vi "Exercise_3-9_Liam_Hubbard.vi"() -> ()   [LabVIEW 2014]
panel:
  in  "Max Wind Speed":dbl
  in  "Current Wind Speed":dbl
  in  "Current Temp":dbl
  in  "Max Temp":dbl
  in  "Min Temp":dbl
  out "Warning Text":string
  out "Warning?":bool
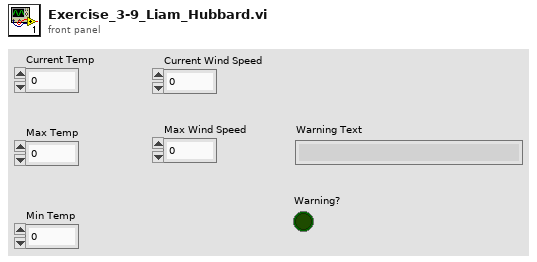
[diagram p1: front panel]
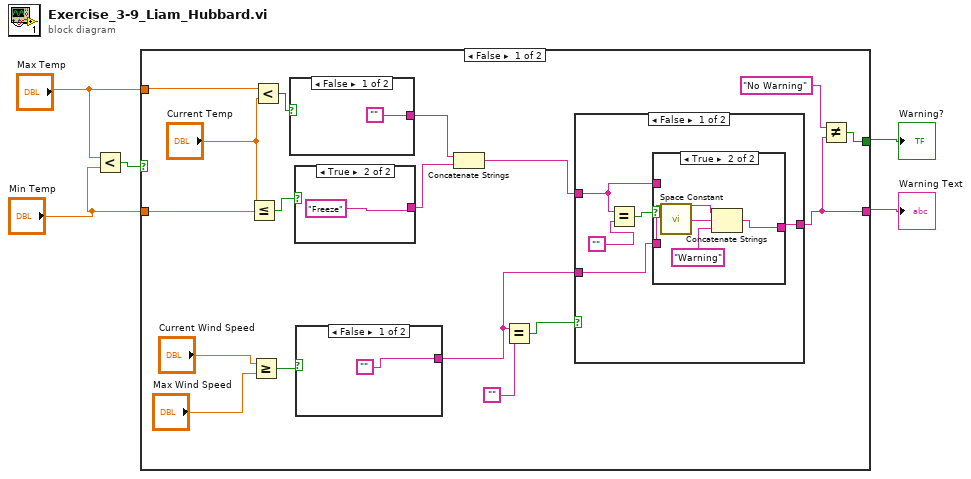
[diagram p0: block diagram]
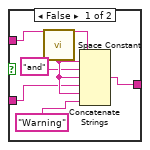
[diagram p2: hidden frame]
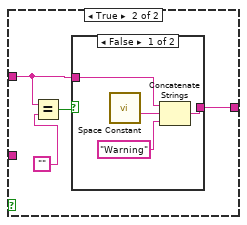
[diagram p3: hidden frame]
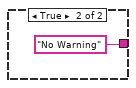
[diagram p4: hidden frame]
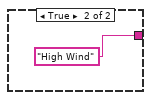
[diagram p5: hidden frame]
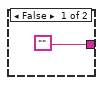
[diagram p6: hidden frame]
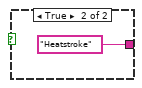
[diagram p7: hidden frame]
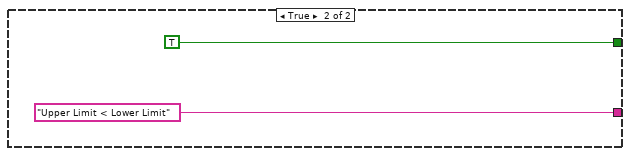
[diagram p8: hidden frame]
diagram:
  n1 = Less?(x="Max Temp", y="Min Temp") -> (x < y?=w3:bool)
  n2 = case shown="False" w3 {
    tunnel: "Max Temp" -> [w21 _]
    tunnel: "Min Temp" -> [w20 _]
    tunnel: [w6 "Upper Limit < Lower Limit"] -> w5
    tunnel: [w8 TRUE] -> w4
    frame False {
      n3 = Less Or Equal?(x="Current Temp", y=w20) -> (x <= y?=w19:bool)
      n4 = Greater Or Equal?(x="Current Wind Speed", y="Max Wind Speed") -> (x >= y?=w17:bool)
      n5 = Less?(x=w21, y="Current Temp") -> (x < y?=w18:bool)
      n6 = case shown="False" w18 {
        tunnel: ["" "Heatstroke" ("t")] -> w13
        frame False {
        }
        frame True {
        }
      }
      n7 = case shown="True" w19 {
        tunnel: ["" "Freeze"] -> w14
        frame False {
        }
        frame True {
        }
      }
      n8 = case shown="False" w17 {
        tunnel: ["" "High Wind"] -> w9
        frame False {
        }
        frame True {
        }
      }
      n9 = Concatenate Strings(w13, w14) -> (w12:string)
      n10 = Equal?(x=w9, y="") -> (x = y?=w11:bool)
      n11 = case shown="False" w11 {
        tunnel: w12 -> [w25 w40]
        tunnel: w9 -> [w23 _]
        tunnel: [w24 w38] -> w6
        frame False {
          n12 = Equal?(x=w25, y="") -> (x = y?=w26:bool)
          n13 = case shown="True" w26 {
            tunnel: w25 -> [w32 _]
            tunnel: [w33 w37] -> w24
            tunnel: w23 -> [w28 w36]
            frame False {
              n14 = call <vilib>:"Space Constant.vi"() -> ("String"=w31:string)
              n15 = Concatenate Strings(w32, w31, "and", w31, w28, w31, "Warning") -> (w33:string)
            }
            frame True {
              n16 = call <vilib>:"Space Constant.vi"() -> ("String"=w34:string)
              n17 = Concatenate Strings(w36, w34, "Warning") -> (w37:string)
            }
          }
        }
        frame True {
          n18 = Equal?(x=w40, y="") -> (x = y?=w41:bool)
          n19 = case shown="False" w41 {
            tunnel: w40 -> [w44 _]
            tunnel: [w45 "No Warning"] -> w38
            frame False {
              n20 = call <vilib>:"Space Constant.vi"() -> ("String"=w43:string)
              n21 = Concatenate Strings(w44, w43, "Warning") -> (w45:string)
            }
            frame True {
            }
          }
        }
      }
      n22 = Not Equal?(x="No Warning", y=w6) -> (x != y?=w8:bool)
    }
    frame True {
    }
  }
  "Warning Text" <- w5
  "Warning?" <- w4
